vi "Update Cycle Count.vi"(8 "error in (no error)":errorcluster, 11 "Spectrum Recorder too in":refnum<class "Spectrum Recorder too.lvclass">) -> (0 "error out":errorcluster, 2 "Cycle count out":i32, 3 "Spectrum Recorder too out":refnum<class "Spectrum Recorder too.lvclass">)   [LabVIEW 2021, in "Spectrum Recorder too.lvclass"]
uses:
  Spectrum Recorder too.lvclass
  C:/GitHub/LabActor/Worker/Worker Actor.lvclass
  Worker/Worker Actor/Worker Actor.lvclass/Worker Actor.ctl
  NHMFL_Core/Libraries/Red Pitaya/RP Core/RP Transceiver/RP Transceiver.lvclass/RP Transceiver.ctl
  Worker/Worker Actor/Read Cycle count.vi
  NHMFL_Core/Libraries/Red Pitaya/RP Core/RP Transceiver/Write Seen last phase word.vi
  Read RP transceiver.vi
  Write RP transceiver.vi
  NHMFL_Core/Libraries/Red Pitaya/RP Core/RP Transceiver/RP Transceiver.lvclass
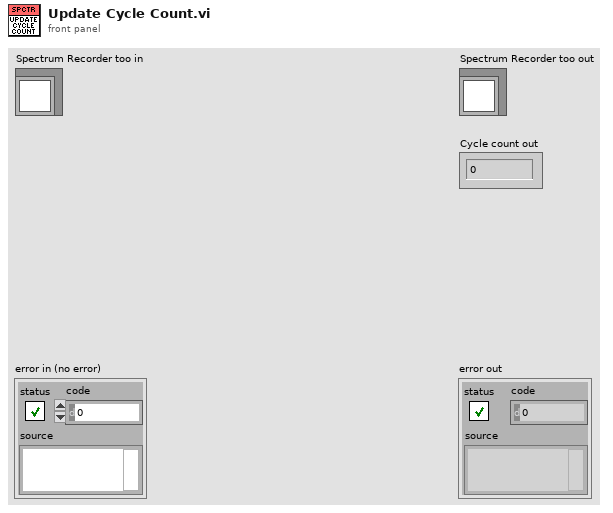
[diagram p1: front panel]
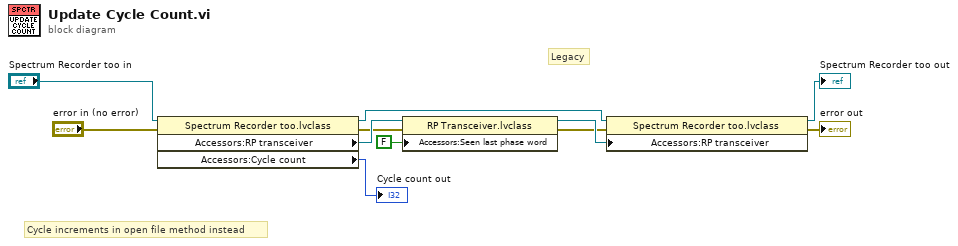
[diagram p0: block diagram]
diagram:
  # "Cycle increments in open file method instead"
  # "Legacy"
  n1 = property class="Spectrum Recorder too.lvclass"(reference="Spectrum Recorder too in", error in="error in (no error)") -> (reference out=w5:refnum<class "Spectrum Recorder too.lvclass">, error out=w8:errorcluster, "Accessors:RP transceiver"=w9:refnum<class "RP Transceiver.lvclass">, "Accessors:Cycle count"=→"Cycle count out":i32)
  n2 = property class="RP Transceiver.lvclass"(reference=w9, error in=w8, "Accessors:Seen last phase word"=FALSE ("Seen last phase word")) -> (reference out=w3:refnum<class "RP Transceiver.lvclass">, error out=w2:errorcluster)
  n3 = property class="Spectrum Recorder too.lvclass"(reference=w5, error in=w2, "Accessors:RP transceiver"=w3) -> (reference out=→"Spectrum Recorder too out":refnum<class "Spectrum Recorder too.lvclass">, error out=→"error out":errorcluster)
